vi "array build.vi"() -> ()   [LabVIEW 2016]
panel:
  out "Appended Array":dbl[][](array[numeric])
  out "Concatenated Array":dbl[](array[numeric])
  in  "Array3":dbl[](array[numeric])
  in  "Array2":dbl[](array[numeric])
  in  "Array1":dbl[](array[numeric])
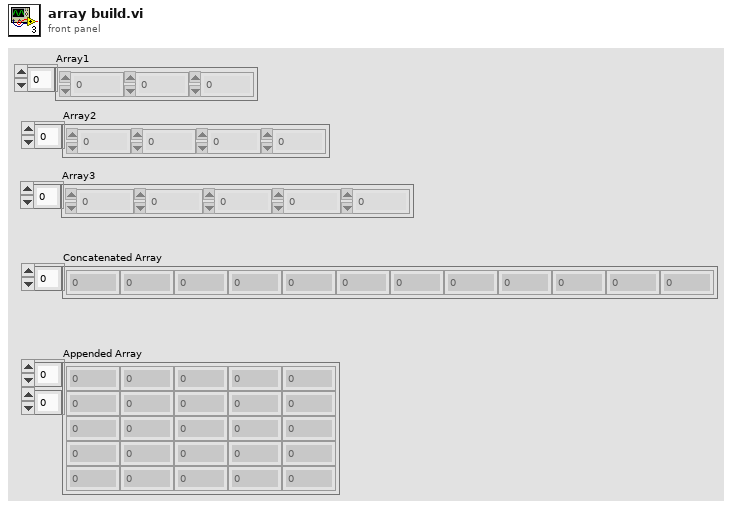
[diagram p1: front panel]
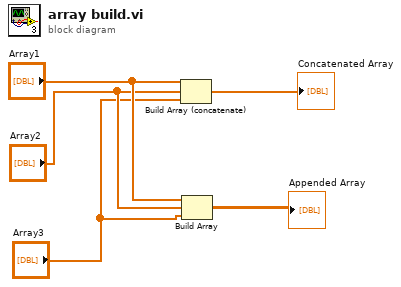
[diagram p0: block diagram]
diagram:
  n1 = Build Array (concatenate)("Array1", "Array2", "Array3") -> (→"Concatenated Array":dbl[])
  n2 = Build Array("Array1", "Array2", "Array3") -> (→"Appended Array":dbl[][])
